vi "TEST.vi"(8 "error in":errorcluster, 11 "Generic Instrument in":refnum<class "Yokogawa WT1600.lvclass">) -> (0 "error out":errorcluster, 3 "Generic Instrument out":refnum<class "Yokogawa WT1600.lvclass">)   [LabVIEW 2013, in "Universal Power Meter.lvlib" / "Yokogawa WT1600.lvlib" / "Yokogawa WT1600.lvclass"]
uses:
  Yokogawa WT1600.lvclass
panel:
  in  "Boolean":bool
  out "resulting string":string
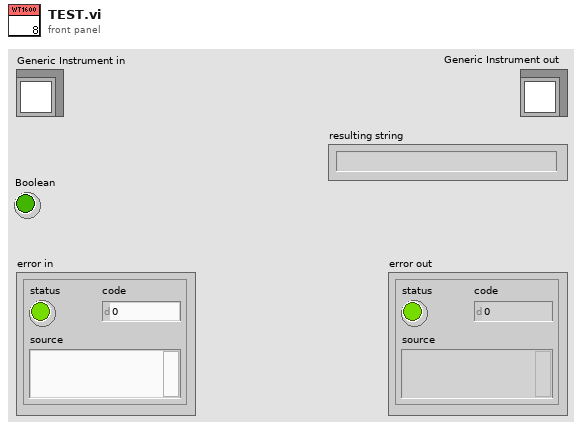
[diagram p1: front panel]
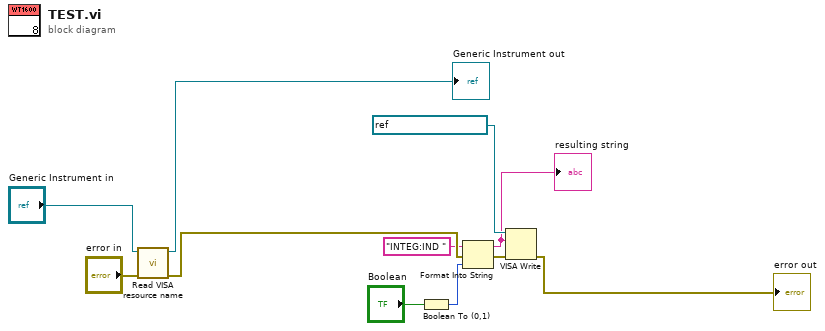
[diagram p0: block diagram]
diagram:
  n1 = call-dynamic "Read VISA resource name.vi"("error in (no error)"="error in", "Generic Instrument in"="Generic Instrument in") -> ("error out"=w11:errorcluster, "Generic Instrument out"=→"Generic Instrument out":refnum<class "Yokogawa WT1600.lvclass">)  [unwired: 7 in, 1 out]
  n2 = Boolean To (0,1)(Boolean="Boolean") -> (0, 1=w2:i16)
  n3 = Format Into String(initial string="INTEG:IND " ("write buffer"), error in=w11, w2) -> (resulting string=w4:string, error out=w6:errorcluster)  [unwired: 1 in]
  "resulting string" <- w4
  n4 = VISA Write(VISA resource name=refnum<visa-resource-name> "GPIB0::10::INSTR", write buffer=w4, error in (no error)=w6) -> (error out=→"error out":errorcluster)  [unwired: 2 out]
